vi "climbmotor.vi"(0 "Cluster 2":T1) -> (7 "Cluster":T1)   [LabVIEW 2018]
uses:
  TypeDefs/Teleop Data Cluster.ctl
  TypeDefs/Joystick Buttons.ctl
panel:
  in  "--":dbl=-0.2 format="%#_13g"
  in  "++":dbl=0.2 format="%#_13g"
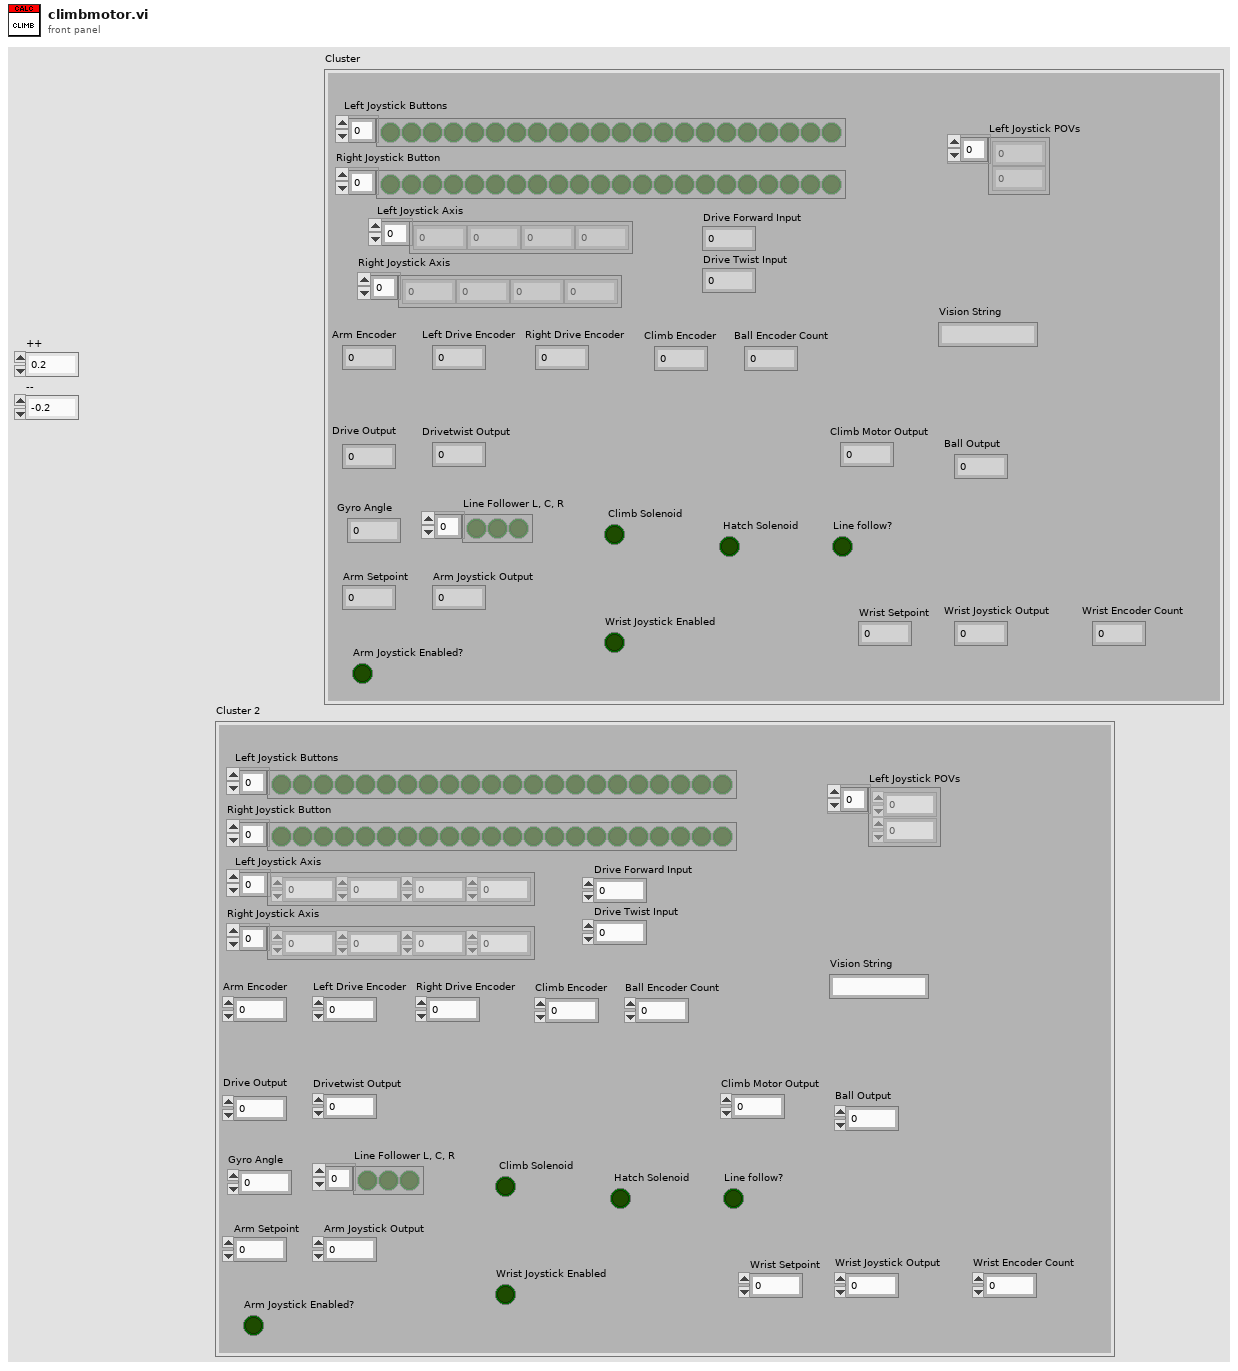
[diagram p1: front panel]
types:
  T1 = typedef "Teleop Data Cluster.ctl" = cluster{"Drive Forward Input ":dbl, "Drive Twist Input":dbl, "Drive Output":dbl, "Drivetwist Output":dbl, "Left Joystick Buttons":bool[], "Left Joystick Axis":dbl[], "Right Joystick Axis":dbl[], "Right Joystick Button":bool[], "Arm Encoder":dbl, "Left Drive Encoder":dbl, "Right Drive Encoder":dbl, "Gyro Angle ":dbl, "Arm Joystick Output  ":dbl, "Line Follower L, C, R ":bool[], "Line follow?":bool, " Climb Solenoid":bool, "Wrist Encoder Count":dbl, "Wrist Joystick Output":dbl, "Ball Encoder Count":dbl, "Ball Output":dbl, "Climb Encoder":dbl, "Climb Motor Output":dbl, " Hatch Solenoid":bool, "Arm Setpoint ":dbl, "Wrist Setpoint ":dbl, "Arm Joystick Enabled?":bool, "Wrist Joystick Enabled":bool, "Vision String":string, "Left Joystick POVs":i16[]}
  T2 = typedef "Joystick Buttons.ctl" = enum16{"Trigger", "Thumb", "Top 3", "Top 4", "Top 5", "Top 6", "Bottom 7", "Bottom 8", "Bottom 9", "Bottom 10", "Bottom 11", "Bottom 12"}
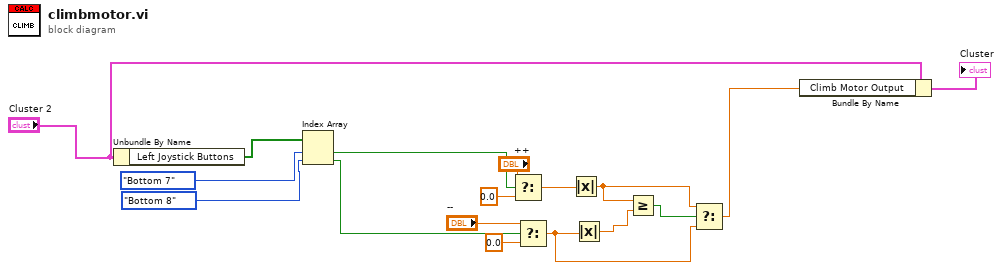
[diagram p0: block diagram]
diagram:
  n1 = Unbundle By Name("Cluster 2") -> ("Left Joystick Buttons"=w12:bool[])
  n2 = Index Array(array=w12, index #1=Joystick_Buttons."Bottom 7" ("Enum"), index #2=Joystick_Buttons."Bottom 8" ("Enum")) -> (element #1=w11:bool, element #2=w10:bool)
  n3 = Select(t="++", s=w11, f=0.0) -> (s? t:f=w6:dbl)
  n4 = Select(t="--", s=w10, f=0.0) -> (s? t:f=w1:dbl)
  n5 = Absolute Value(x=w6) -> (abs(x)=w4:dbl)
  n6 = Absolute Value(x=w1) -> (abs(x)=w3:dbl)
  n7 = Greater Or Equal?(x=w4, y=w3) -> (x >= y?=w5:bool)
  n8 = Select(t=w4, s=w5, f=w1) -> (s? t:f=w2:dbl)
  n9 = Bundle By Name(cluster="Cluster 2", "Climb Motor Output"=w2) -> (→"Cluster":T1)
